vi "36 GPS String Manipulation (x64-2018).vi"(10 "CPU Time In":dbl format="%#.6f", 11 "Input String":string) -> (3 "GPS Time Code":string)   [LabVIEW 2017]
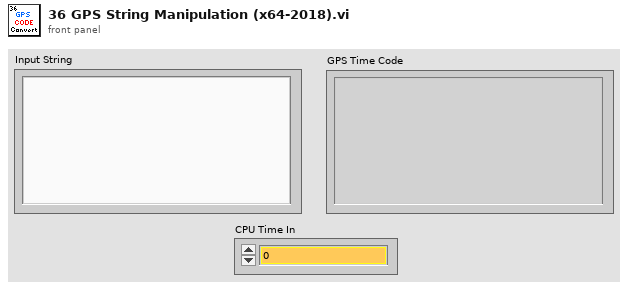
[diagram p1: front panel]
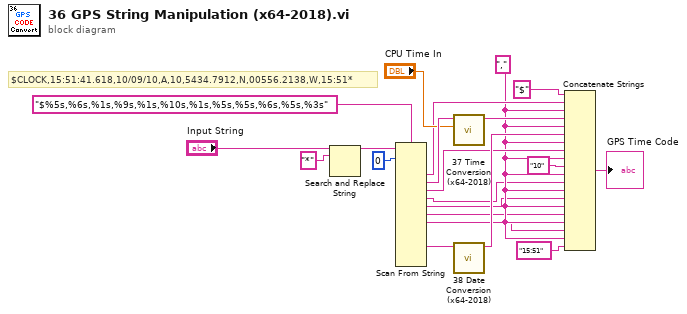
[diagram p0: block diagram]
diagram:
  w7 = ","
  # "$CLOCK,15:51:41.618,10/09/10,A,10,5434.7912,N,00556.2138,W,15:51*"
  n1 = Search and Replace String(input string="Input String", search string="*") -> (result string=w9:string)  [unwired: 6 in, 3 out]
  n2 = Scan From String(format string="$%5s,%6s,%1s,%9s,%1s,%10s,%1s,%5s,%5s,%6s,%5s,%3s", input string=w9, initial scan location=0) -> (output 1=w14:string, output 2=w18:string, output 3=w10:string, output 4=w3:string, output 5=w4:string, output 6=w5:string, output 7=w6:string, output 10=w12:string)  [unwired: 17 in, 3 out]
  n3 = call "37 Time Conversion (x64-2018).vi"("CPU Time In"="CPU Time In", "Time In"=w18) -> ("Time Out"=w13:string)  [unwired: 9 in]
  n4 = call "38 Date Conversion (x64-2018).vi"("Date In"=w12) -> ("Date Out"=w11:string)  [unwired: 10 in]
  n5 = Concatenate Strings("$", w14, w7, w13, w7, w11, w7, w10, w7, "10", w7, w3, w7, w4, w7, w5, w7, w6, w7, "15:51") -> (→"GPS Time Code":string)
